vi "OpenKlubmodulCSV.vi"(11 "CSV String":string) -> (3 "CSV Data":string[][](array[string]))   [LabVIEW 2018]
doc: "Convert Klubmodul CSV file to String array.\n\nKåre Juul Kirkegaard"
uses:
  <vilib>/Utility/error.llb/whitespace.ctl
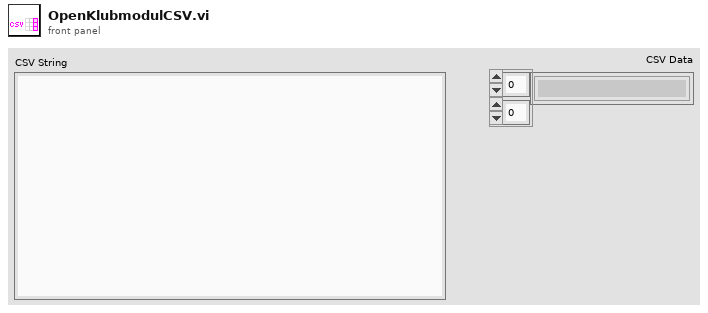
[diagram p1: front panel]
types:
  T1 = typedef "whitespace.ctl" = u16
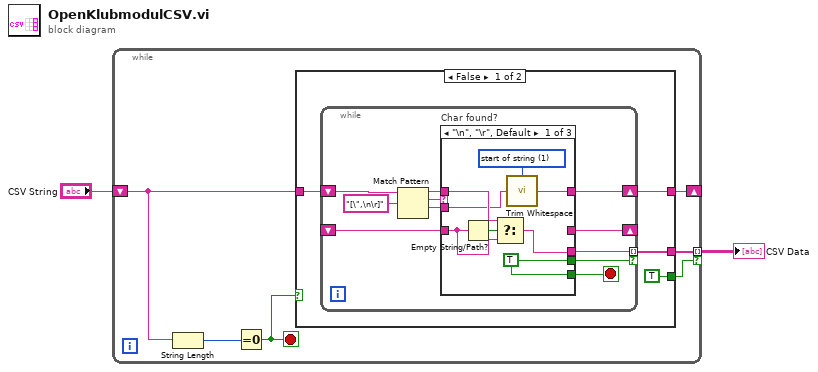
[diagram p0: block diagram]
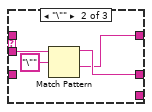
[diagram p2: hidden frame]
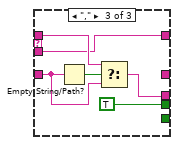
[diagram p3: hidden frame]
diagram:
  n1 = while {
    tunnel: [w8] -> w2 mode=indexing if=w3
    shift-right: [w7] -> _
    shift-left: "CSV String" -> [w6]
    stop <- w4 stop-if-true
    n2 = String Length(string=w6) -> (length=w5:i32)
    n3 = Equal To 0?(x=w5) -> (x = 0?=w4:bool)
    n4 = case shown="False" w4 {
      tunnel: [w12 _] -> w8
      tunnel: [w11 w42] -> w7
      tunnel: w6 -> [w10 w42]
      tunnel: [TRUE _] -> w3
      frame False {
        n5 = while {
          shift-right: [w14] -> w11
          shift-left: w10 -> [w23]
          shift-right: [w18] -> _
          shift-left: _ -> [w17]
          tunnel: [w16] -> w12 mode=indexing if=w15
          stop <- w13 stop-if-true
          n6 = Match Pattern(string=w23, regular expression="[\",\n\r]") -> (before substring=w19:string, match substring=w21:string, after substring=w20:string)  [unwired: 1 in, 1 out]
          n7 = case "Char found?" shown="\"\\n\", \"\\r\", Default" w21 {
            tunnel: w20 -> [w25 w33 w36]
            tunnel: w19 -> [w30 _ w40]
            tunnel: [_ w34 _] -> w18
            tunnel: w17 -> [w29 _ w39]
            tunnel: [w28 _ w38] -> w16
            tunnel: [w27 _ TRUE] -> w15
            tunnel: [w26 w32 w36] -> w14
            tunnel: [w27 _ _] -> w13
            frame "\n", "\r", Default {
              w24 = T1 1 items=["both", "start of string", "end of string"] ("location (both)")
              w27 = TRUE
              n8 = Empty String/Path?(string/path=w29) -> (empty?=w31:bool)
              n9 = Select(t=w30, s=w31, f=w29) -> (s? t:f=w28:string)
              n10 = call <vilib>:"Trim Whitespace.vi"("string"=w25, "location (both)"=w24) -> ("trimmed string"=w26:string)
            }
            frame "\"" {
              n11 = Match Pattern(string=w33, regular expression="\"") -> (before substring=w34:string, after substring=w32:string)  [unwired: 1 in, 2 out]
            }
            frame "," {
              n12 = Empty String/Path?(string/path=w39) -> (empty?=w41:bool)
              n13 = Select(t=w40, s=w41, f=w39) -> (s? t:f=w38:string)
            }
          }
        }
      }
      frame True {
      }
    }
  }
  "CSV Data" <- w2
